vi "TimeLoop.vi"() -> ()   [LabVIEW 2017]
uses:
  <vilib>/Utility/file.llb/Read Delimited Spreadsheet (I64).vi
panel:
  out "z 2":i64
  out "y 2":i64
  out "x 2":i64
  out "all rows":i64[][](array[numeric])
  out "z":i64
  out "y":i64
  out "x":i64
  out "Time":i32
  out "Speed Z":i32
  out "Speed X":i32
  out "Speed Y":i32
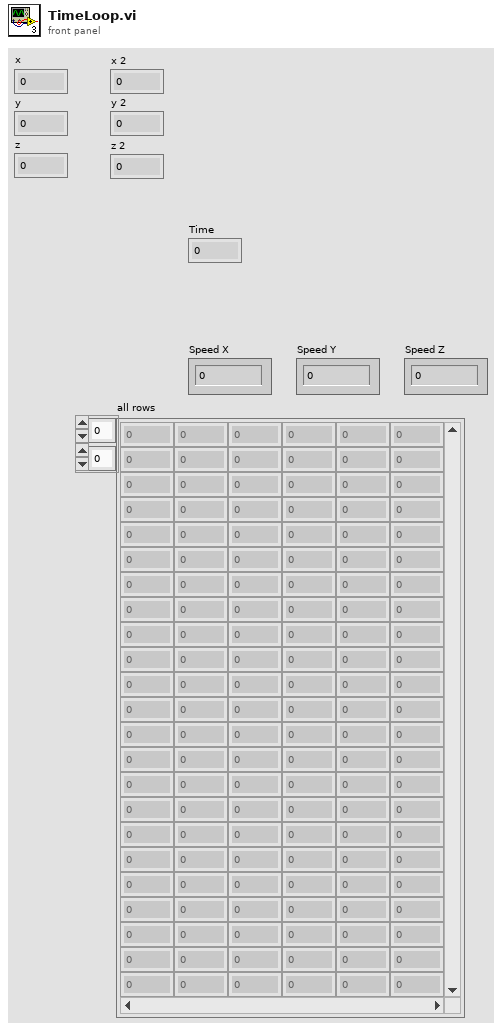
[diagram p1: front panel]
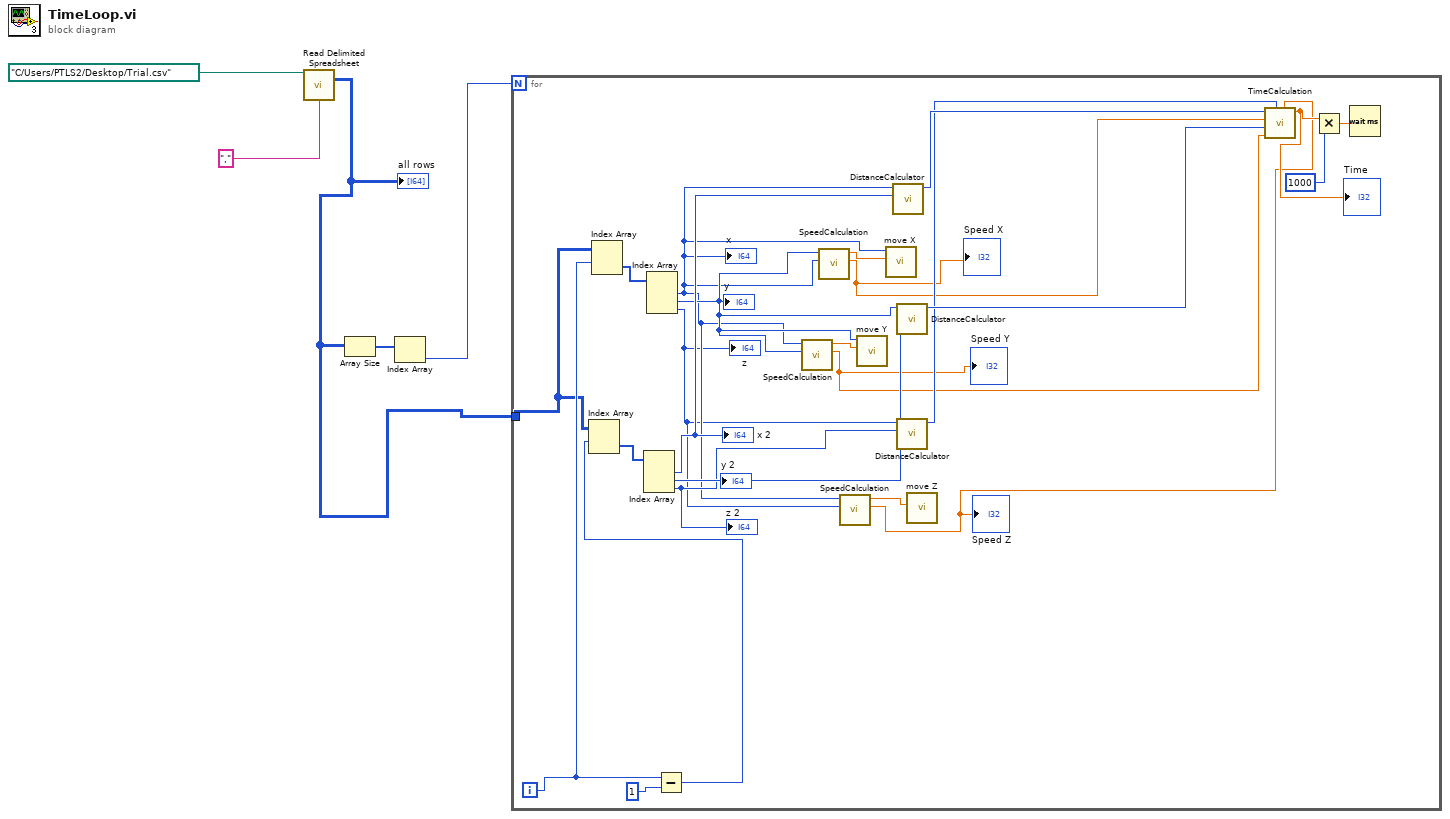
[diagram p0: block diagram]
diagram:
  n1 = call-poly <vilib>:"Read Delimited Spreadsheet.vi"("file path (dialog if empty)"=path "C:/Users/PTLS2/Desktop/Trial.csv", "delimiter (\\t)"="," ("delimiter (\\t)")) -> ("all rows"=w3:i64[][])  [unwired: 8 in, 5 out]
  "all rows" <- w3
  n2 = Array Size(array=w3) -> (size(s)=w5:i32[])
  n3 = Index Array(array=w5) -> (element=w4:i32)  [unwired: 1 in]
  n4 = for {
    N: w4 -> [_]
    tunnel: w3 -> [w19]
    i -> [w22]
    n5 = Index Array(array=w19, index (row)=w22) -> (element=w18:i64[])  [unwired: 1 in]
    n6 = Index Array(array=w18) -> (element #1=w10:i64, element #2=w12:i64, element #3=w9:i64)  [unwired: 3 in]
    "x" <- w10
    "y" <- w12
    "z" <- w9
    n7 = Subtract(x=w22, y=1) -> (x-y=w20:i32)
    n8 = Index Array(array=w19, index (row)=w20) -> (element=w21:i64[])  [unwired: 1 in]
    n9 = Index Array(array=w21) -> (element #1=w17:i64, element #2=w16:i64, element #3=w15:i64)  [unwired: 3 in]
    "x 2" <- w17
    "y 2" <- w16
    "z 2" <- w15
    n10 = call "SpeedCalculation.vi"("Axis1"=w12, "Axis2"=w10) -> ("Speed mm/s"=w7:dbl, "Speed for card"=w13:dbl)  [unwired: 8 in]
    "Speed Y" <- w7
    n11 = call "SpeedCalculation.vi"("Axis1"=w10, "Axis2"=w12) -> ("Speed mm/s"=w8:dbl, "Speed for card"=w14:dbl)  [unwired: 8 in]
    "Speed X" <- w8
    n12 = call "SpeedCalculation.vi"("Axis1"=w9, "Axis2"=w10) -> ("Speed mm/s"=w6:dbl, "Speed for card"=w11:dbl)  [unwired: 8 in]
    "Speed Z" <- w6
    n13 = call "move Y.vi"("Y Speed"=w13, "y mm"=w12) -> ()  [unwired: 10 in]
    n14 = call "move X.vi"("Speed X"=w14, "x mm"=w10) -> ()  [unwired: 10 in]
    n15 = call "DistanceCalculator.vi"("Number2"=w17, "Number1"=w10) -> ("Distance"=w25:i32)  [unwired: 9 in]
    n16 = call "DistanceCalculator.vi"("Number2"=w16, "Number1"=w12) -> ("Distance"=w24:i32)  [unwired: 9 in]
    n17 = call "DistanceCalculator.vi"("Number2"=w15, "Number1"=w9) -> ("Distance"=w23:i32)  [unwired: 9 in]
    n18 = call "move Z.vi"("Y Speed"=w11) -> ()  [unwired: 11 in]
    n19 = call "TimeCalculation.vi"("Speed Z"=w6, "Position Z"=w23, "SpeedY"=w7, "Y Position"=w24, "Speed X"=w8, "X Position"=w25) -> ("Time"=w27:dbl)  [unwired: 5 in]
    "Time" <- w27
    n20 = Multiply(x=w27, y=1000) -> (x*y=w29:dbl)
    n21 = Wait (ms)(milliseconds to wait=w29) -> ()  [unwired: 1 out]
  }
